vi "dfd_Build TFs from Lattice Coefficients.vi"(8 "error in (no error)":errorcluster, 11 "am":dbl[](array[numeric])) -> (0 "error out":errorcluster, 1 "gain":dbl, 2 "h1":dbl[](array[numeric]), 3 "h0":dbl[](array[numeric]))   [LabVIEW 2017, in "NI_DigFilter_FilterBank.lvlib"]
uses:
  <vilib>/addons/Digital Filter Design/NI_DigFilter_FilterBank.lvlib
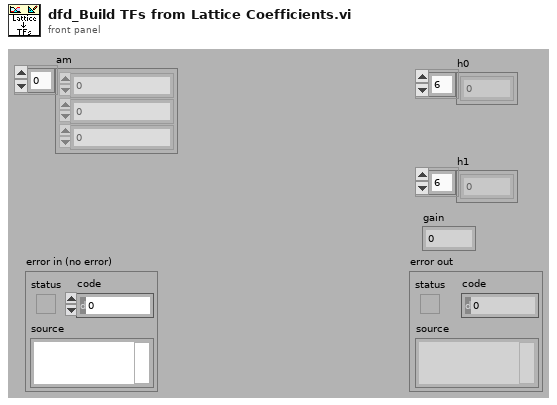
[diagram p1: front panel]
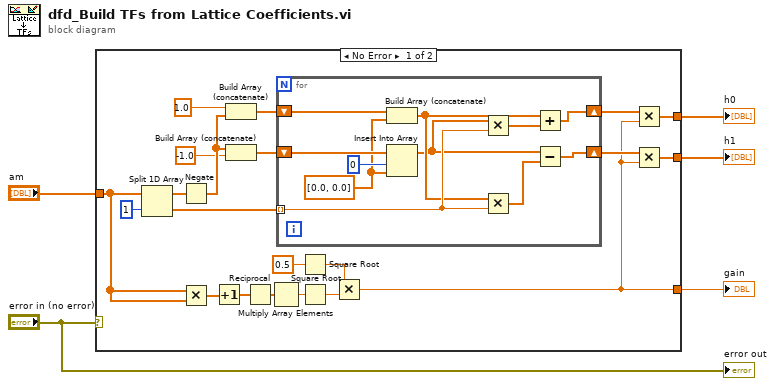
[diagram p0: block diagram]
diagram:
  n1 = case shown="No Error" "error in (no error)" {
    tunnel: [w20 _] -> w5
    tunnel: [w19 _] -> w4
    tunnel: "am" -> [w7 _]
    tunnel: [w6 _] -> w2
    frame No Error {
      n2 = Split 1D Array(array=w7, index=1) -> (first subarray=w23:dbl[], second subarray=w26:dbl[])
      n3 = Negate(x=w23) -> (-x=w18:dbl[])
      n4 = Multiply(x=w7, y=w7) -> (x*y=w9:dbl[])
      n5 = Increment(x=w9) -> (x+1=w10:dbl[])
      n6 = Build Array (concatenate)(1.0, w18) -> (w24:dbl[])
      n7 = Build Array (concatenate)(w18, -1.0) -> (w21:dbl[])
      n8 = Reciprocal(x=w10) -> (1/x=w8:dbl[])
      n9 = Multiply Array Elements(1:w8) -> (0:w14:dbl)
      n10 = for {
        tunnel: w26 -> [w33] mode=indexing
        shift-right: [w34] -> w16
        shift-left: w24 -> [w27]
        shift-right: [w32] -> w15
        shift-left: w21 -> [w37]
        w28 = dbl[] [0.0, 0.0]
        n11 = Build Array (concatenate)(w27, w28) -> (w31:dbl[])
        n12 = Insert Into Array(array=w37, index=0, new element=w28) -> (w29:dbl[])
        n13 = Multiply(x=w29, y=w33) -> (x*y=w35:dbl[])
        n14 = Multiply(x=w31, y=w33) -> (x*y=w30:dbl[])
        n15 = Add(x=w31, y=w35) -> (x+y=w34:dbl[])
        n16 = Subtract(x=w29, y=w30) -> (x-y=w32:dbl[])
      }
      n17 = Square Root(x=0.5) -> (sqrt(x)=w11:dbl)
      n18 = Square Root(x=w14) -> (sqrt(x)=w13:dbl)
      n19 = Multiply(x=w11, y=w13) -> (x*y=w6:dbl)
      n20 = Multiply(x=w16, y=w6) -> (x*y=w20:dbl[])
      n21 = Multiply(x=w15, y=w6) -> (x*y=w19:dbl[])
    }
    frame Error {
    }
  }
  "h0" <- w5
  "h1" <- w4
  "gain" <- w2
  "error out" <- "error in (no error)"
